vi "CreatePublicEvents.vi"(8 "error in (no error)":errorcluster, 11 "SynchIO.USB4431":refnum<class "SynchIO.USB4431.lvclass">) -> (0 "error out":errorcluster, 3 "SynchIO.USB4431 out":refnum<class "SynchIO.USB4431.lvclass">)   [LabVIEW 2016, in "SynchIO.USB4431.lvclass"]
doc: "---------------------------------------------------------------\nJKI State Machine Objects™\nhttp://jki.net/state-machine-objects/\nCopyright (C) 2005-2015, JKI <info@jki.net>\nALL RIGHTS RESERVEDJKI State Machine Objects (SMO) 1.0.0.5\nJKI - JKI\nCopyright (c) 2016, JKI"
uses:
  SynchIO.USB4431.lvclass
  Typedefs/DataChanged--EventData--Cluster.ctl
  SynchIO.USB4431.lvclass/SynchIO.USB4431.ctl
  Typedefs/PublicEvents--SynchIO.USB4431.Initialize.ctl
  SynchIO/SynchIO.lvclass
panel:
  # "For instructions on how to use the JKI State Machine Objects, examples and video tutorials, visit:\nhttp://jki.net/state-machine-objects/\n\nJKI State Machine Objects™\nhttp://jki.net/state-machine-objects/\nCopyright (C) 2005-2015, JKI <info@jki.net>\nALL RIGHTS RESERVED"
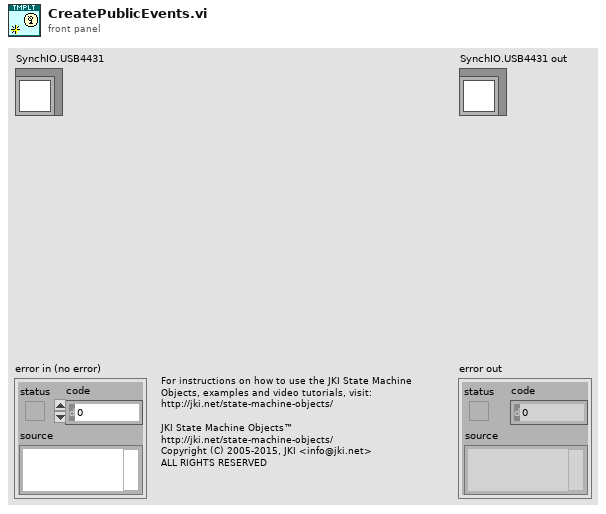
[diagram p1: front panel]
types:
  T1 = typedef "SynchIO.USB4431.lvclass/DataChanged--EventData--Cluster.ctl" = cluster{"Timestamp":timestamp, "Old Value":string, "New Value":string}
  T2 = typedef "SynchIO.USB4431.lvclass/PrivateData--Ref.ctl" = refnum<data-value>
  T3 = typedef "SynchIO.USB4431.lvclass/PublicEvents--SynchIO.USB4431.Initialize.ctl" = bool
  T4 = typedef "SynchIO.USB4431.lvclass/PrivateData--Cluster.ctl" = cluster{"Configuration":T5, "Public Events":T6, "Protected Events":T7, "Data":string, "Private Events":T8}
  T5 = typedef "SynchIO.USB4431.lvclass/Configuration--Cluster.ctl" = cluster{"Suffix":string}
  T6 = typedef "SynchIO.USB4431.lvclass/PublicEvents--Cluster.ctl" = cluster{"Data Changed":refnum<user-event>, "Initialize":refnum<user-event>}
  T7 = typedef "SynchIO.USB4431.lvclass/ProtectedEvents--Cluster.ctl" = cluster{"API_Template":refnum<user-event>}
  T8 = typedef "SynchIO.USB4431.lvclass/PrivateEvents--Cluster.ctl" = cluster{"Initialize":refnum<user-event>, "Init":refnum<user-event>, "Init-Event":refnum<user-event>}
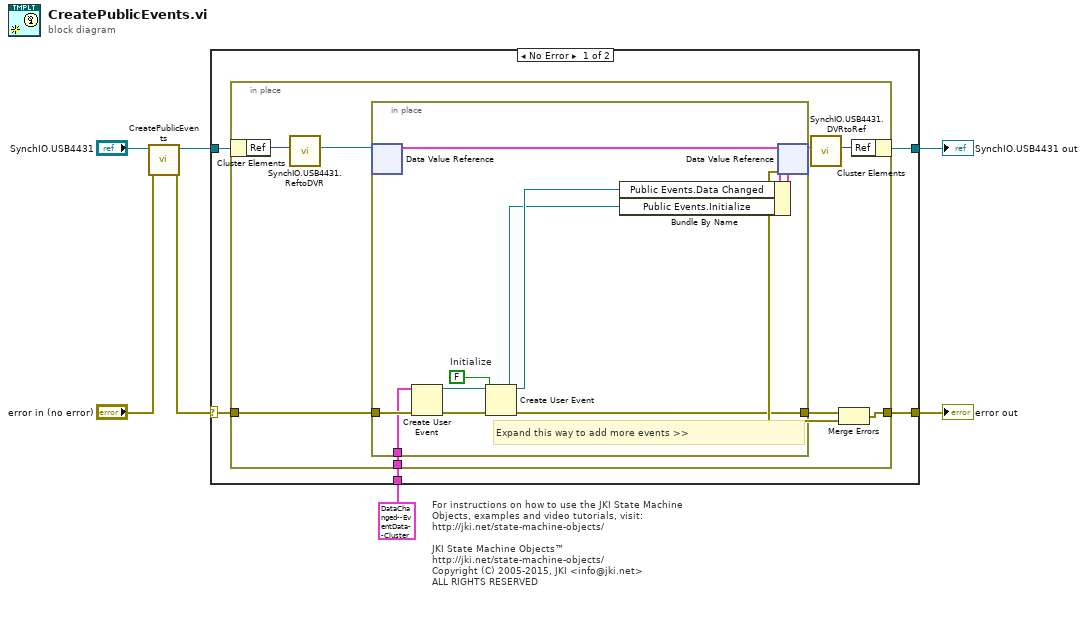
[diagram p0: block diagram]
diagram:
  # "For instructions on how to use the JKI State Machine Objects, examples and video tutorials, visit:\nhttp://jki.net/state-machine-objects/\n\nJKI State Machine Objects™\nhttp://jki.net/state-machine-objects/\nCopyright (C) 2005-2015, JKI <info@jki.net>\nALL RIGHTS RESERVED"
  n1 = call-parent "CreatePublicEvents.vi"("error in (no error)"="error in (no error)", "SynchIO"="SynchIO.USB4431") -> ("error out"=w1:errorcluster, "SynchIO out"=w3:refnum<class "SynchIO.USB4431.lvclass">)  [unwired: 8 in]
  n2 = case shown="No Error" w1 {
    selector: w1 -> [w10 w32]
    tunnel: [w9 w32] -> w6
    tunnel: [w11 w31] -> w7
    tunnel: w3 -> [w12 w31]
    tunnel: T1 {"Timestamp"=timestamp(0 s since 1904-01-01), "Old Value"="", "New Value"=""} ("Data In Event Data") -> [w8 _]
    frame No Error {
      n3 = in-place {
        in-place-border: w10 -> [w21]
        in-place-border: [w18] -> w9
        in-place-border: w8 -> [w17]
        n4 = in-place-cluster #1(w12) -> ("Ref"=w16:u32)
        n5 = call "SynchIO.USB4431.ReftoDVR.vi"("Ref"=w16) -> ("Ref"=w15:T2)  [unwired: 10 in]
        n6 = in-place {
          in-place-border: w21 -> [w27]
          in-place-border: [w24] -> w20
          in-place-border: w17 -> [w26]
          w23 = T3 FALSE  # Initialize
          # "Expand this way to add more events >>"
          n7 = in-place-dvr #2(w15) -> (w29:T4)  [unwired: 1 out]
          n8 = Create User Event(user event datatype=w26, error in=w27) -> (user event=w25:refnum<user-event>, error out=w28:errorcluster)
          n9 = Create User Event(user event datatype=w23, error in=w28) -> (user event=w22:refnum<user-event>, error out=w24:errorcluster)
          n10 = Bundle By Name(cluster=w29, "Public Events.Data Changed"=w25, "Public Events.Initialize"=w22) -> (w30:T4)
          n11 = in-place-dvr #2(w30) -> (w14:T2, w19:errorcluster)
        }
        n12 = call "SynchIO.USB4431.DVRtoRef.vi"("Ref"=w14) -> ("Ref"=w13:u32)  [unwired: 10 in]
        n13 = Merge Errors(w20, w19) -> (w18:errorcluster)
        n14 = in-place-cluster #1("Ref"=w13) -> (w11:refnum<class "SynchIO.USB4431.lvclass">)
      }
    }
    frame Error {
    }
  }
  "error out" <- w6
  "SynchIO.USB4431 out" <- w7
